vi "setExposureTime.vi"(8 "error in (no error)":errorcluster, 10 "exposure_time_s":dbl, 11 "Camera in":refnum<class "Camera.lvclass">) -> (0 "error out":errorcluster, 3 "Camera out":refnum<class "Camera.lvclass">)   [LabVIEW 2019, in "Camera.lvclass"]
doc: "Sets the exposure time of the camera, in seconds. The values for the underlying pco.sdk function PCO_SetDelayExposureTime.vi will be calculated automatically."
uses:
  Camera.lvclass
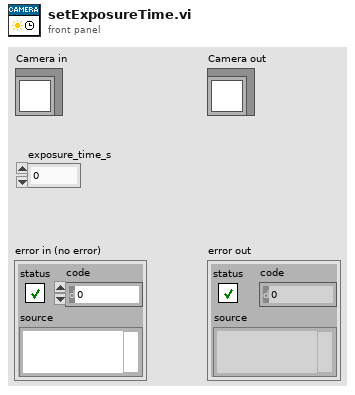
[diagram p1: front panel]
types:
  T1 = typedef "Camera.lvclass/binning.ctl" = cluster{"vert":u16, "horz":u16, "mode":u16}
  T2 = cluster{"exposure_time_s":dbl, "delay_time_s":dbl, "roi":cluster{"x0":u64, "y0":u64, "x1":u64, "y1":u64}, "timestamp_mode":u16, "pixelrate":u32, "conversion_factor":sgl, "trigger_mode":u16, "acquire_mode":u16, "acquire_sequence_number":u32, "metadata_mode":u16, "noisefilter_mode":u16, "pixel_format":u32, "binning":T1, "auto_exposure":cluster{"region":u16, "min_exposure_s":dbl, "max_exposure_s":dbl}}
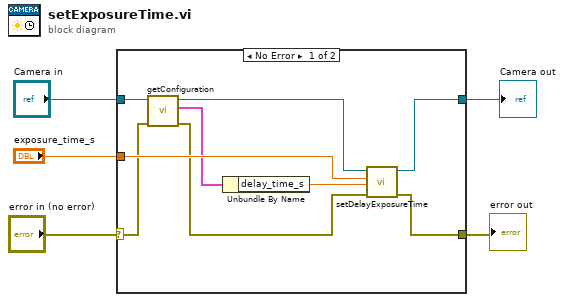
[diagram p0: block diagram]
diagram:
  n1 = case shown="No Error" "error in (no error)" {
    selector: "error in (no error)" -> [w10 w16]
    tunnel: [w13 w16] -> w5
    tunnel: [w12 w15] -> w4
    tunnel: "Camera in" -> [w11 w15]
    tunnel: "exposure_time_s" -> [w14 _]
    frame No Error {
      n2 = call-dynamic "getConfiguration.vi"("error in (no error)"=w10, "Camera in"=w11) -> ("error out"=w9:errorcluster, "configuration"=w8:T2, "Camera out"=w6:refnum<class "Camera.lvclass">)  [unwired: 7 in]
      n3 = Unbundle By Name(w8) -> ("delay_time_s"=w7:dbl)
      n4 = call-dynamic "setDelayExposureTime.vi"("error in (no error)"=w9, "delay_time_s"=w7, "exposure_time_s"=w14, "Camera in"=w6) -> ("error out"=w13:errorcluster, "Camera out"=w12:refnum<class "Camera.lvclass">)  [unwired: 6 in]
    }
    frame Error {
    }
  }
  "error out" <- w5
  "Camera out" <- w4
